vi "Show Cursors.vi"(6 "Cursor Options":T1={"font"={"Font Name"="Arial", "Size"=14, "Strikeout?"=FALSE, "Italic?"=FALSE, "Underline?"=FALSE, "Outline?"=FALSE, "Shadow?"=FALSE, "Bold?"=FALSE}, "size"=1, "Timestamp"=enum."at TOP", "Vertical Line?"=FALSE, "Horizontal Line?"=FALSE, "alignment(left, top)"={"horizontal"=enum."center", "vertical"=enum."center"}, "TextFormat"="%2$.2f\\n\\n%1$s", "time format (%H:%M:%S)"="%H:%M%:S"} {"size" min=1 max=50}, 8 "error in (no error)":errorcluster, 9 "Coords":T2, 10 "XY Graph":refnum<vi>, 11 "input picture":picture) -> (0 "error out":errorcluster, 3 "output picture":picture)   [LabVIEW 2020, in "Graph Extensions.lvlib"]
doc: "Shows real time cursors overlayed in a graph, using just one mouse move event case. The options for the cursors can be highly customized to set up a unique cursor style.\n\nUsage: Place this inside an event structure on any XY graph, in the \"Mouse Move\" event case. Set the options as an input cluster to override the defaults. The output picture control would typically be connected to the XY Graph's \"PlotImages.Front\" property item.\n\nCursor Options\n<b>Horizontal Line?</b> - Draws a horizontal line to intersect each plot\n<b>Verticle Line?</b> - Draws a verticle line at the mouse location to highlight the cursor location (typically on the time scale)\n<b>Timestamp</b> - Sets where to display the timestamp (if you want it at the top or bottom) Used best with the verticle line turned on.\n<b>Font</b> - Setup the font for displaying the cursor text\n<b>Alignment</b> - Sets the alignment options for the text relative to the cursor point\n<b>TextFormat</b> - Sets the text display format at the cursor points to show. Three input parameters are available for the text, which can be accessed using parameter numbers.\ninputs: \n1$ - Timestamp at cursor locations\n2$ - Value of the plot\n3$ - Name of the plot\n\nExamples: $2$.2f\\n\\n%1$s\nThis shows the value of the plot with 2 decimal places. A blank line, then the name of the plot"
uses:
  Documents/WeChat Files/zps501304/FileStorage/File/2020-11/Graph-Extensions-LabVIEW-master/source/Graph Extensions.lvlib
  <vilib>/Utility/miscctls.llb/LVPoint32TypeDef.ctl
  Documents/WeChat Files/zps501304/FileStorage/File/2020-11/Graph-Extensions-LabVIEW-master/source/controls/CursorOptions.ctl
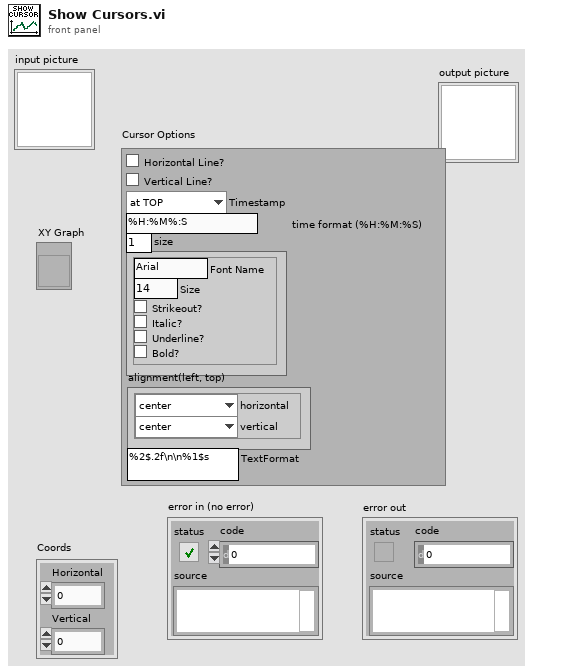
[diagram p1: front panel]
types:
  T1 = typedef "Graph Extensions.lvlib/CursorOptions.ctl" = cluster{"font":cluster{"Font Name":string, "Size":i16, "Strikeout?":bool, "Italic?":bool, "Underline?":bool, "Outline?":bool, "Shadow?":bool, "Bold?":bool}, "size":i16, "Timestamp":enum16{"at TOP", "at BOTTOM", "none"}, "Vertical Line?":bool, "Horizontal Line?":bool, "alignment(left, top)":cluster{"horizontal":enum16{"left", "center", "right"}, "vertical":enum16{"top", "center", "bottom"}}, "TextFormat":string, "time format (%H:%M:%S)":string}
  T2 = typedef "LVPoint32TypeDef.ctl" = cluster{"Horizontal":i32, "Vertical":i32}
  T3 = enum16{"User-specified Font", "Application Font", "System Font", "Dialog Font"}
  T4 = cluster{"horizontal":enum16{"left", "center", "right"}, "vertical":enum16{"top", "center", "bottom"}}
  T5 = cluster{"Font Name":string, "Size":i16, "Strikeout?":bool, "Italic?":bool, "Underline?":bool, "Outline?":bool, "Shadow?":bool, "Bold?":bool}
  T6 = typedef "LVRectTypeDef.ctl" = cluster{"Left":i16, "Top":i16, "Right":i16, "Bottom":i16}
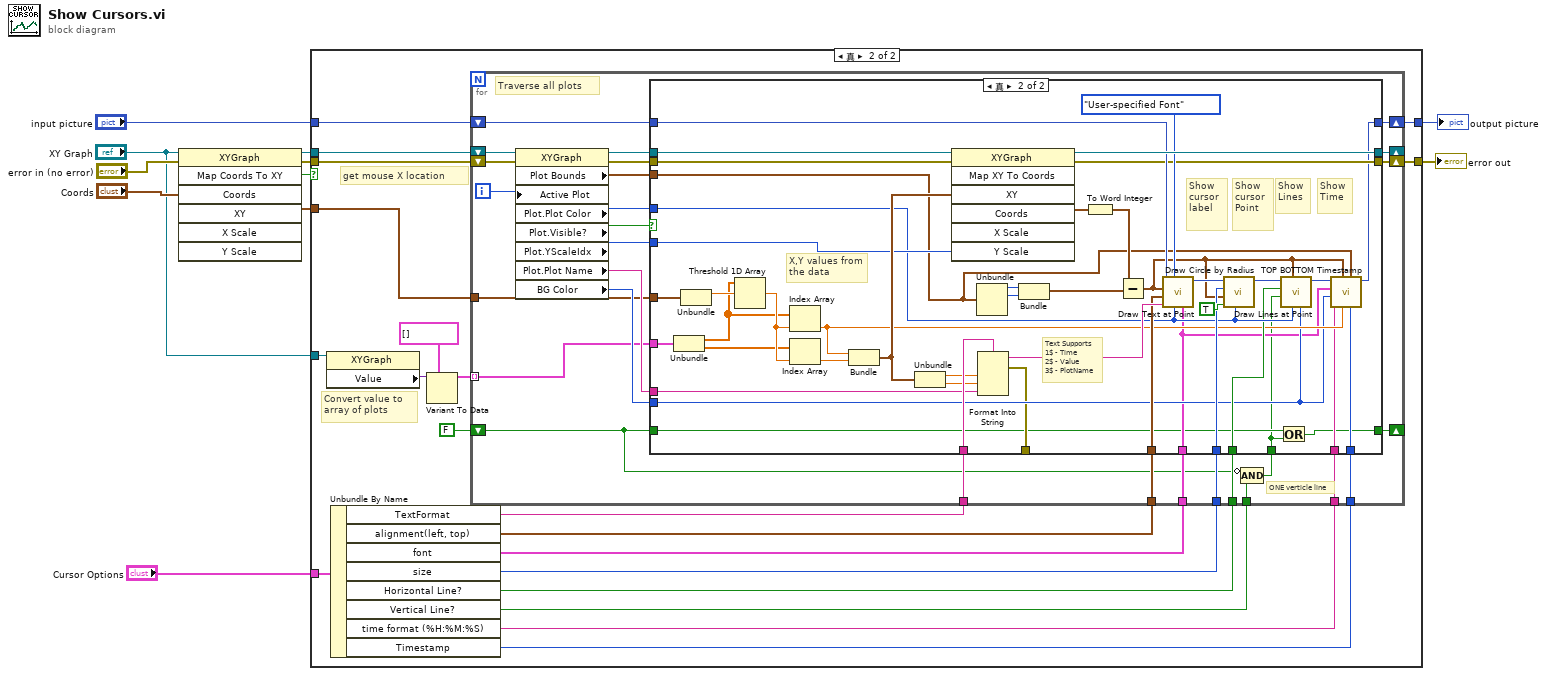
[diagram p0: block diagram]
diagram:
  n1 = invoke on="Invoke Node" class="XYGraph" method="Map Coords To XY"(reference="XY Graph", error in="error in (no error)", "Coords"="Coords") -> (reference out=w8:refnum<vi>, error out=w7:errorcluster, "Map Coords To XY"=w10:bool, "XY"=w11:cluster{"X":dbl, "Y":dbl})  [unwired: 4 in, 3 out]
  n2 = case shown="真" w10 {
    tunnel: w11 -> [_ w32]
    tunnel: w8 -> [_ w33]
    tunnel: [w12 w31] -> w3
    tunnel: w7 -> [w13 w30]
    tunnel: [w13 w29] -> w6
    tunnel: "input picture" -> [w12 w28]
    tunnel: "Cursor Options" -> [_ w20]
    tunnel: "XY Graph" -> [_ w17]
    frame False {
      # "not in plot area.  clear the image"
    }
    frame True {
      # "Convert value to array of plots"
      # "get mouse X location"
      n3 = property class="XYGraph"(reference=w17) -> ("Value"=w16:variant)  [unwired: 1 in, 2 out]
      n4 = Unbundle By Name(w20) -> ("TextFormat"=w27:string, "alignment(left, top)"=w26:T4, "font"=w25:T5, "size"=w24:i16, "Horizontal Line?"=w23:bool, "Vertical Line?"=w22:bool, "time format (%H:%M:%S)"=w15:string, "Timestamp"=w21:enum16{"at TOP", "at BOTTOM", "none"})
      n5 = Variant To Data(type=cluster{dbl[], dbl[]}[] [], Variant=w16) -> (data=w19:cluster{dbl[], dbl[]}[])  [unwired: 1 in, 1 out]
      n6 = for {
        tunnel: w19 -> [w37] mode=indexing
        shift-right: [w60] -> _
        shift-left: w33 -> [w58]
        tunnel: w32 -> [w38]
        shift-right: [w56] -> w31
        shift-left: w28 -> [w59]
        shift-right: [w51] -> w29
        shift-left: w30 -> [w53]
        tunnel: w24 -> [w49]
        tunnel: w26 -> [w48]
        tunnel: w25 -> [w47]
        tunnel: w27 -> [w46]
        tunnel: w23 -> [w45]
        tunnel: w22 -> [w42]
        tunnel: w21 -> [w40]
        tunnel: w15 -> [w36]
        shift-right: [w34] -> _
        shift-left: FALSE -> [w35]
        i -> [w44]
        # "Traverse all plots"
        # "ONE verticle line"
        n7 = property on="Property Node" class="XYGraph"(reference=w58, error in=w53, "Active Plot"=w44) -> (reference out=w57:refnum<vi>, error out=w52:errorcluster, "Plot Bounds"=w61:T6, "Plot.Plot Color"=w55:u32, "Plot.Visible?"=w54:bool, "Plot.YScaleIdx"=w50:u32, "Plot.Plot Name"=w41:string, "BG Color"=w39:u32)
        n8 = Compound Arithmetic op=AND(invert w35, w42) -> (w43:bool)
        n9 = case shown="真" w54 {
          tunnel: w61 -> [_ w74]
          tunnel: [w65 w105] -> w60
          tunnel: w37 -> [_ w100]
          tunnel: w38 -> [_ w99]
          tunnel: w59 -> [w64 w98]
          tunnel: w57 -> [w65 w95]
          tunnel: [w64 w79] -> w56
          tunnel: w55 -> [_ w84]
          tunnel: w52 -> [w63 w91]
          tunnel: [w63 w90] -> w51
          tunnel: w50 -> [_ w89]
          tunnel: w49 -> [_ w88]
          tunnel: w48 -> [_ w87]
          tunnel: w47 -> [_ w72]
          tunnel: w46 -> [_ w86]
          tunnel: w45 -> [_ w83]
          tunnel: w43 -> [_ w67]
          tunnel: w41 -> [_ w80]
          tunnel: w40 -> [_ w76]
          tunnel: w39 -> [_ w73]
          tunnel: [_ w70] -> _
          tunnel: w36 -> [_ w69]
          tunnel: w35 -> [w62 w68]
          tunnel: [w62 w66] -> w34
          frame False {
            # "plot is not visible, so don't show the cursor for it."
          }
          frame True {
            # "Show\nTime"
            # "Show\nLines"
            # "Show\ncursor\nPoint"
            # "Show\ncursor\nlabel"
            # "Text Supports\n1$ - Time\n2$ - Value\n3$ - PlotName"
            # "X,Y values from the data"
            n10 = Unbundle(w100) -> (w71:dbl[], w102:dbl[])
            n11 = Unbundle(w99) -> ("X"=w101:dbl)  [unwired: 1 out]
            n12 = Threshold 1D Array(2:w101, 3:w71) -> (0:w103:dbl)  [unwired: 1 in]
            n13 = Index Array(array=w71, index=w103) -> (element=w77:dbl)
            n14 = Index Array(array=w102, index=w103) -> (element=w104:dbl)
            n15 = Bundle("X"=w77, "X"=w104) -> (w97:cluster{"X":dbl, "X":dbl})  [unwired: 1 in]
            n16 = Unbundle(w97) -> ("X"=w82:dbl, "X"=w81:dbl)
            n17 = invoke on="Invoke Node" class="XYGraph" method="Map XY To Coords"(reference=w95, error in=w91, "XY"=w97, "Y Scale"=w89) -> (reference out=w105:refnum<vi>, error out=w90:errorcluster, "Coords"=w110:T2)  [unwired: 3 in, 4 out]
            n18 = Unbundle(w74) -> ("Left"=w108:i16, "Top"=w109:i16)  [unwired: 2 out]
            n19 = Format Into String(format string=w86, w82, w81, w80) -> (resulting string=w96:string, error out=w70:errorcluster)  [unwired: 2 in]
            n20 = Bundle("Left"=w108, "Top"=w109) -> (w106:cluster{"Left":i16, "Top":i16})  [unwired: 1 in]
            n21 = To Word Integer(number=w110) -> (16bit integer=w107:cluster{"Horizontal":i16, "Vertical":i16})
            n22 = Subtract(x=w107, y=w106) -> (x-y=w75:cluster{i16, i16})
            n23 = call <vilib>:"Draw Text at Point.vi"("[user-specified font]"=w72, "text color(black)"=w84, "desired font(Application)"=T3."User-specified Font", "text"=w96, "alignment(left, top)"=w87, "origin"=w75, "picture"=w98) -> ("new picture"=w94:picture)  [unwired: 3 in, 1 out]
            n24 = call <vilib>:"Draw Circle by Radius.vi"("color(black)"=w84, "fill?(F)"=TRUE, "pixel center"=w75, "radius"=w88, "picture"=w94) -> ("new picture"=w85:picture)  [unwired: 6 in]
            n25 = Or(x=w68, y=w67) -> (x .or. y?=w66:bool)
            n26 = call "Draw Lines at Point.vi"("GraphBGK"=w73, "color(black)"=w84, "pixel center"=w75, "Vertical Line?"=w67, "Horizontal Line?"=w83, "new picture in"=w85) -> ("new picture out"=w78:picture)  [unwired: 5 in]
            n27 = call "TOP BOTTOM Timestamp.vi"("Format"=w76, "Rect"=w74, "Timestamp"=w77, "pixel center"=w75, "time format (%H:%M:%S)"=w69, "GraphBGK"=w73, "font"=w72, "new picture in"=w78) -> ("new picture out"=w79:picture)  [unwired: 3 in]
          }
        }
      }
    }
  }
  "error out" <- w6
  "output picture" <- w3
